vi "JSR GUI.vi"(8 "error in (no error)":errorcluster, 10 "JSR Complete":T1={"JSR Pulse Settings"={"Damping"=59, "Pulse Energy Level"=2, "Pulser Impedance"=0, "Pulser Voltage (V)"=100}, "JSR Receive Settings"={"Receiver Mode"=0, "High Pass Filter"=5000, "Low Pass Filter"=50, "Gain (dB)"=50}, "JSR Trigger Settings"={"External Trigger Limit"=0, "Trigger Source"=1, "PRF (Hz)"=1.75}} {"JSR Trigger Settings"."PRF (Hz)" items=["100 Hz"=0.1, "200 Hz"=0.2, "400 Hz"=0.4, "600 Hz"=0.6, "800 Hz"=0.8, "1000 Hz"=1.0, "1250 Hz"=1.25, "1500 Hz"=1.5, "1750 Hz"=1.75, "2000 Hz"=2.0, "2500 Hz"=2.5, "3000 Hz"=3.0, "3500 Hz"=3.5, "4000 Hz"=4.0, "4500 Hz"=4.5, "5000 Hz"=5.0]; "JSR Trigger Settings"."Trigger Source" items=["Internal", "External"]; "JSR Trigger Settings"."External Trigger Limit" items=["No Limit", "5 kHz"]; "JSR Receive Settings"."Gain (dB)" min=-13 max=66 step=1; "JSR Receive Settings"."Low Pass Filter" items=["5 MHz"=5, "10 MHz"=10, "15 MHz"=15, "22.5 MHz"=22, "35 MHz"=35, "50 MHz"=50]; "JSR Receive Settings"."High Pass Filter" items=["DC"=0, "1 MHz"=1000, "2.5 MHz"=2500, "5 MHz"=5000, "7.5 MHz"=7500, "12.5 MHz"=12500]; "JSR Receive Settings"."Receiver Mode" items=["Echo", "Through"]; "JSR Pulse Settings"."Pulser Voltage (V)" items=["100"=100, "125"=125, "150"=150, "175"=175, "200"=200, "225"=225, "250"=250, "275"=275, "300"=300, "325"=325, "350"=350, "375"=375, "400"=400, "425"=425, "450"=450, "475"=475]; "JSR Pulse Settings"."Pulser Impedance" items=["High z", "Low z"]; "JSR Pulse Settings"."Pulse Energy Level" items=["0 (Minimum)", "1", "2", "3 (Maximum)"]; "JSR Pulse Settings"."Damping" items=["331 Ohms"=331, "198 Ohms"=198, "142 Ohms"=142, "110 Ohms"=110, "92 Ohms"=92, "77 Ohms"=77, "67 Ohms"=67, "59 Ohms"=59, "52 Ohms"=52, "47 Ohms"=47, "43 Ohms"=43, "39 Ohms"=39, "37 Ohms"=37, "34 Ohms"=34, "32 Ohms"=32, "30 Ohms"=30]}, 11 "JSR VISA":refnum<visa-resource-name>) -> (0 "error out":errorcluster, 2 "JSR Complete Out":T1={"JSR Pulse Settings"={"Damping"=59, "Pulse Energy Level"=2, "Pulser Impedance"=0, "Pulser Voltage (V)"=100}, "JSR Receive Settings"={"Receiver Mode"=0, "High Pass Filter"=5000, "Low Pass Filter"=50, "Gain (dB)"=50}, "JSR Trigger Settings"={"External Trigger Limit"=0, "Trigger Source"=1, "PRF (Hz)"=1.75}} {"JSR Trigger Settings"."PRF (Hz)" items=["100 Hz"=0.1, "200 Hz"=0.2, "400 Hz"=0.4, "600 Hz"=0.6, "800 Hz"=0.8, "1000 Hz"=1.0, "1250 Hz"=1.25, "1500 Hz"=1.5, "1750 Hz"=1.75, "2000 Hz"=2.0, "2500 Hz"=2.5, "3000 Hz"=3.0, "3500 Hz"=3.5, "4000 Hz"=4.0, "4500 Hz"=4.5, "5000 Hz"=5.0]; "JSR Trigger Settings"."Trigger Source" items=["Internal", "External"]; "JSR Trigger Settings"."External Trigger Limit" items=["No Limit", "5 kHz"]; "JSR Receive Settings"."Gain (dB)" min=-13 max=66 step=1; "JSR Receive Settings"."Low Pass Filter" items=["5 MHz"=5, "10 MHz"=10, "15 MHz"=15, "22.5 MHz"=22, "35 MHz"=35, "50 MHz"=50]; "JSR Receive Settings"."High Pass Filter" items=["DC"=0, "1 MHz"=1000, "2.5 MHz"=2500, "5 MHz"=5000, "7.5 MHz"=7500, "12.5 MHz"=12500]; "JSR Receive Settings"."Receiver Mode" items=["Echo", "Through"]; "JSR Pulse Settings"."Pulser Voltage (V)" items=["100"=100, "125"=125, "150"=150, "175"=175, "200"=200, "225"=225, "250"=250, "275"=275, "300"=300, "325"=325, "350"=350, "375"=375, "400"=400, "425"=425, "450"=450, "475"=475]; "JSR Pulse Settings"."Pulser Impedance" items=["High z", "Low z"]; "JSR Pulse Settings"."Pulse Energy Level" items=["0 (Minimum)", "1", "2", "3 (Maximum)"]; "JSR Pulse Settings"."Damping" items=["331 Ohms"=331, "198 Ohms"=198, "142 Ohms"=142, "110 Ohms"=110, "92 Ohms"=92, "77 Ohms"=77, "67 Ohms"=67, "59 Ohms"=59, "52 Ohms"=52, "47 Ohms"=47, "43 Ohms"=43, "39 Ohms"=39, "37 Ohms"=37, "34 Ohms"=34, "32 Ohms"=32, "30 Ohms"=30]}, 3 "JSR VISA Out":refnum<visa-resource-name>)   [LabVIEW 2022 SP3]
uses:
  Controls/JSR Pulse.ctl
  Controls/Damping.ctl
  Controls/Energy.ctl
  Controls/Z.ctl
  Controls/Volt.ctl
  Controls/JSR Recieve.ctl
  Controls/Mode.ctl
  Controls/HPF.ctl
  Controls/LPF.ctl
  Controls/Gain.ctl
  Controls/JSR Trigger.ctl
  Controls/Trig Limit.ctl
  Controls/Trig Source.ctl
  Controls/PRF.ctl
  Controls/JSR Complete.ctl
  PulserGlobals.vi
panel:
  in  "Exit":bool
  in  "JSR Trigger Settings":T12={"External Trigger Limit"=0, "Trigger Source"=1, "PRF (Hz)"=0.6} {"PRF (Hz)" items=["100 Hz"=0.1, "200 Hz"=0.2, "400 Hz"=0.4, "600 Hz"=0.6, "800 Hz"=0.8, "1000 Hz"=1.0, "1250 Hz"=1.25, "1500 Hz"=1.5, "1750 Hz"=1.75, "2000 Hz"=2.0, "2500 Hz"=2.5, "3000 Hz"=3.0, "3500 Hz"=3.5, "4000 Hz"=4.0, "4500 Hz"=4.5, "5000 Hz"=5.0]; "Trigger Source" items=["Internal", "External"]; "External Trigger Limit" items=["No Limit", "5 kHz"]}
  in  "JSR Receive Settings":T7={"Receiver Mode"=0, "High Pass Filter"=5000, "Low Pass Filter"=50, "Gain (dB)"=50} {"Gain (dB)" min=-13 max=66 step=1; "Low Pass Filter" items=["5 MHz"=5, "10 MHz"=10, "15 MHz"=15, "22.5 MHz"=22, "35 MHz"=35, "50 MHz"=50]; "High Pass Filter" items=["DC"=0, "1 MHz"=1000, "2.5 MHz"=2500, "5 MHz"=5000, "7.5 MHz"=7500, "12.5 MHz"=12500]; "Receiver Mode" items=["Echo", "Through"]}
  in  "JSR Pulse Settings":T2={"Damping"=43, "Pulse Energy Level"=3, "Pulser Impedance"=0, "Pulser Voltage (V)"=100} {"Pulser Voltage (V)" items=["100"=100, "125"=125, "150"=150, "175"=175, "200"=200, "225"=225, "250"=250, "275"=275, "300"=300, "325"=325, "350"=350, "375"=375, "400"=400, "425"=425, "450"=450, "475"=475]; "Pulser Impedance" items=["High z", "Low z"]; "Pulse Energy Level" items=["0 (Minimum)", "1", "2", "3 (Maximum)"]; "Damping" items=["331 Ohms"=331, "198 Ohms"=198, "142 Ohms"=142, "110 Ohms"=110, "92 Ohms"=92, "77 Ohms"=77, "67 Ohms"=67, "59 Ohms"=59, "52 Ohms"=52, "47 Ohms"=47, "43 Ohms"=43, "39 Ohms"=39, "37 Ohms"=37, "34 Ohms"=34, "32 Ohms"=32, "30 Ohms"=30]}
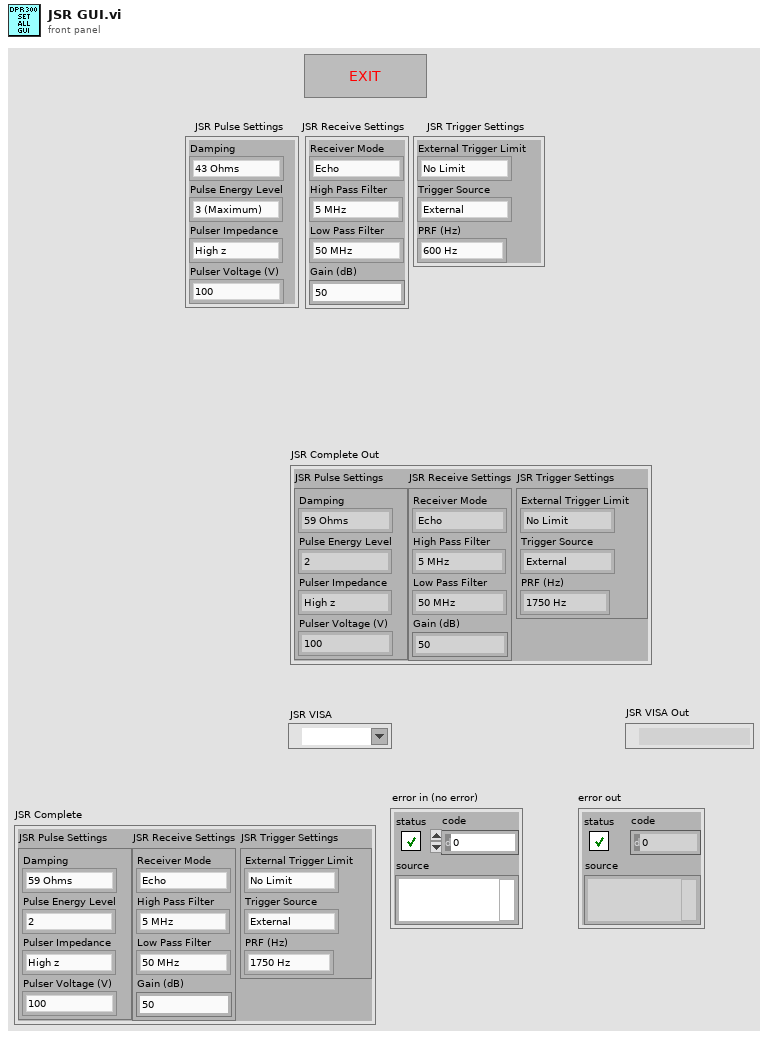
[diagram p1: front panel]
types:
  T1 = typedef "JSR Complete.ctl" = cluster{"JSR Pulse Settings":T2, "JSR Receive Settings":T7, "JSR Trigger Settings":T12}
  T2 = typedef "JSR Pulse.ctl" = cluster{"Damping":T3, "Pulse Energy Level":T4, "Pulser Impedance":T5, "Pulser Voltage (V)":T6}
  T3 = typedef "Damping.ctl" = i16
  T4 = typedef "Energy.ctl" = u16
  T5 = typedef "Z.ctl" = u16
  T6 = typedef "Volt.ctl" = i16
  T7 = typedef "JSR Recieve.ctl" = cluster{"Receiver Mode":T8, "High Pass Filter":T9, "Low Pass Filter":T10, "Gain (dB)":T11}
  T8 = typedef "Mode.ctl" = i8
  T9 = typedef "HPF.ctl" = u16
  T10 = typedef "LPF.ctl" = u16
  T11 = typedef "Gain.ctl" = i8
  T12 = typedef "JSR Trigger.ctl" = cluster{"External Trigger Limit":T13, "Trigger Source":T14, "PRF (Hz)":T15}
  T13 = typedef "Trig Limit.ctl" = i8
  T14 = typedef "Trig Source.ctl" = i8
  T15 = typedef "PRF.ctl" = dbl
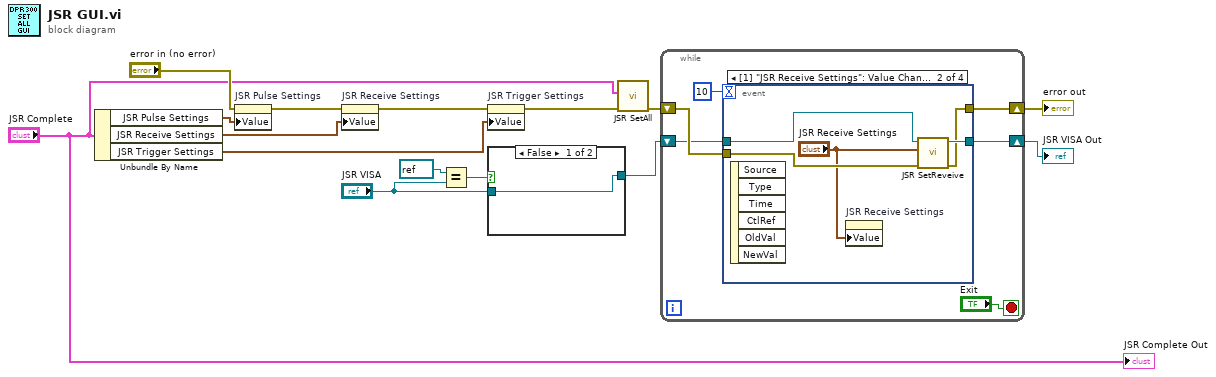
[diagram p0: block diagram]
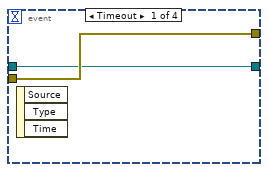
[diagram p2: hidden frame]
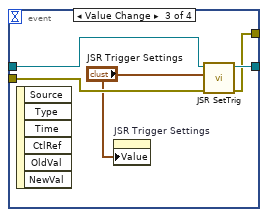
[diagram p3: hidden frame]
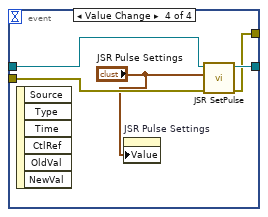
[diagram p4: hidden frame]
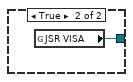
[diagram p5: hidden frame]
diagram:
  n1 = Unbundle By Name("JSR Complete") -> ("JSR Pulse Settings"=w7:T2, "JSR Receive Settings"=w8:T7, "JSR Trigger Settings"=w6:T12)
  n2 = property on="JSR Pulse Settings" class="Clust (strict)"(error in="error in (no error)", "Value"=w7) -> (error out=w4:errorcluster)  [unwired: 1 in, 1 out]
  n3 = property on="JSR Receive Settings" class="Clust (strict)"(error in=w4, "Value"=w8) -> (error out=w3:errorcluster)  [unwired: 1 in, 1 out]
  n4 = Equal?(x=refnum<visa-resource-name> refnum, y="JSR VISA") -> (x = y?=w10:bool)
  n5 = property on="JSR Trigger Settings" class="Clust (strict)"(error in=w3, "Value"=w6) -> (error out=w2:errorcluster)  [unwired: 1 in, 1 out]
  n6 = case shown="False" w10 {
    tunnel: [w16 w17] -> w13
    tunnel: "JSR VISA" -> [w16 _]
    frame False {
    }
    frame True {
      n7 = global read "PulserGlobals.vi" "JSR VISA"() -> (w17:refnum<visa-resource-name>)
    }
  }
  n8 = call "JSR SetAll.vi"("error in (no error)"=w2, "JSR Complete"="JSR Complete") -> ("error out"=w9:errorcluster)  [unwired: 8 in, 1 out]
  n9 = while {
    shift-right: [w21] -> w14
    shift-left: w9 -> [w23]
    shift-right: [w22] -> w15
    shift-left: w13 -> [w20]
    stop <- "Exit" stop-if-true
    n10 = event shown="[1] \"JSR Receive Settings\": Value Change" {
      selector: _ -> [_ _ _ _]
      dyn-events: _ -> [_ _ _ _]
      timeout: 10 -> [_ _ _ _]
      tunnel: w23 -> [w25 w30 w35 w40]
      tunnel: [w24 w29 w33 w39] -> w22
      tunnel: [w25 w28 w32 w38] -> w21
      tunnel: w20 -> [w24 w27 w34 w37]
      event Timeout {
        n11 = event-data() -> ()  [unwired: 1 in, 3 out]
      }
      event Value Change {
        n12 = event-data() -> ()  [unwired: 1 in, 6 out]
        n13 = property on="JSR Receive Settings" class="Clust (strict)"("Value"="JSR Receive Settings") -> ()  [unwired: 2 in, 2 out]
        n14 = call "JSR SetReveive.vi"("error in (no error)"=w30, "JSR Receive Settings"="JSR Receive Settings", "VISA Refnum in"=w27) -> ("error out"=w28:errorcluster, "VISA Refnum out"=w29:refnum<visa-resource-name>)  [unwired: 7 in]
      }
      event Value Change {
        n15 = event-data() -> ()  [unwired: 1 in, 6 out]
        n16 = property on="JSR Trigger Settings" class="Clust (strict)"("Value"="JSR Trigger Settings") -> ()  [unwired: 2 in, 2 out]
        n17 = call "JSR SetTrig.vi"("error in (no error)"=w35, "JSR Trigger Settings"="JSR Trigger Settings", "VISA Refnum in"=w34) -> ("error out"=w32:errorcluster, "VISA Refnum out"=w33:refnum<visa-resource-name>)  [unwired: 7 in]
      }
      event Value Change {
        n18 = event-data() -> ()  [unwired: 1 in, 6 out]
        n19 = property on="JSR Pulse Settings" class="Clust (strict)"("Value"="JSR Pulse Settings") -> ()  [unwired: 2 in, 2 out]
        n20 = call "JSR SetPulse.vi"("error in (no error)"=w40, "JSR Pulse Settings"="JSR Pulse Settings", "VISA Refnum in"=w37) -> ("error out"=w38:errorcluster, "VISA Refnum out"=w39:refnum<visa-resource-name>)  [unwired: 7 in]
      }
    }
  }
  "error out" <- w14
  "JSR VISA Out" <- w15
  "JSR Complete Out" <- "JSR Complete"
